vi "Create Plugin Project.vi"(8 "error in":errorcluster, 9 "Custom Device Name":string, 11 "CDEW_MetaDataObj in":refnum<class "NIVS_CDEW_MetaDataObj.lvclass">) -> (0 "error out":errorcluster, 3 "CDEW_MetaDataObj out":refnum<class "NIVS_CDEW_MetaDataObj.lvclass">)   [LabVIEW 2026, in "NIVS_CDEW_MetaDataObj.lvclass"]
uses:
  NIVS_CDEW_MetaDataObj.lvclass
  Types/PluginProjectToolStates.ctl
  NIVS_CDEW_MetaDataObj.lvclass/NIVS_CDEW_MetaDataObj.ctl
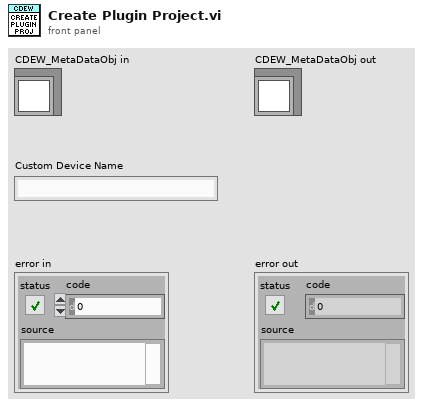
[diagram p1: front panel]
types:
  T1 = typedef "NIVS_CDEW_MetaDataObj.lvclass/PluginProjectToolStates.ctl" = enum16{"CopyAndRenamePluginLVLIB", "CopyAndRenameDeploymentHooksLVLIB", "UpdateProject"}
  T2 = typedef "NIVS_CDEW_MetaDataObj.lvclass/Execution Modes.ctl" = enum16{"Inline HW Interface (Inline-Async API)", "Inline HW Interface", "Inline Timing and Sync"}
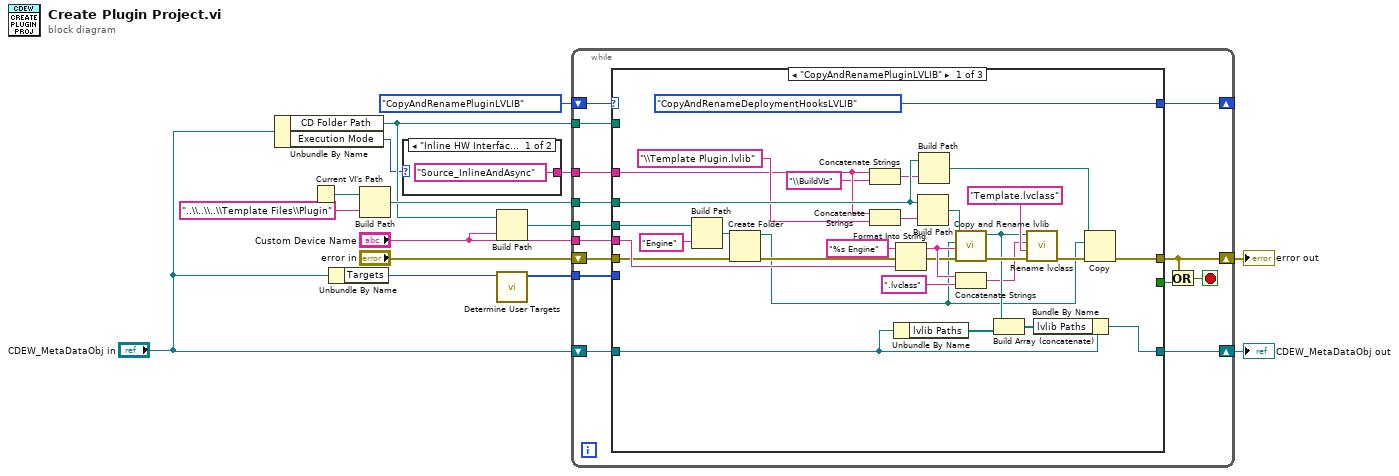
[diagram p0: block diagram]
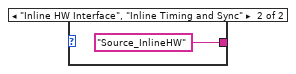
[diagram p2: hidden frame]
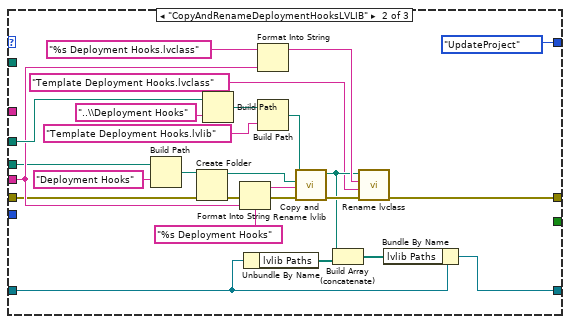
[diagram p3: hidden frame]
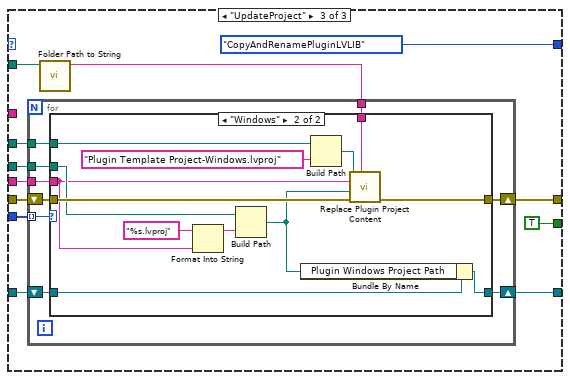
[diagram p4: hidden frame]
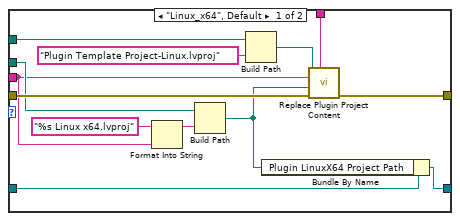
[diagram p5: hidden frame]
diagram:
  n1 = Unbundle By Name("CDEW_MetaDataObj in") -> ("CD Folder Path"=w4:path, "Execution Mode"=w3:T2)
  n2 = Current VI's Path() -> (path=w14:path)
  n3 = Unbundle By Name("CDEW_MetaDataObj in") -> ("Targets"=w5:enum16{"Linux_x64", "Windows", "Both"})
  n4 = Build Path(base path=w14, name or relative path="..\\..\\..\\Template Files\\Plugin") -> (appended path=w12:path)
  n5 = case shown="\"Inline HW Interface (Inline-Async API)\", Default" w3 {
    tunnel: ["Source_InlineAndAsync" ("string") "Source_InlineHW" ("string")] -> w9
    frame "Inline HW Interface (Inline-Async API)", Default {
    }
    frame "Inline HW Interface", "Inline Timing and Sync" {
    }
  }
  n6 = Build Path(base path=w4, name or relative path="Custom Device Name") -> (appended path=w7:path)
  n7 = call "Determine User Targets.vi"("Targets"=w5) -> ("User Configured Targets"=w6:enum16{"Linux_x64", "Windows", "Both"}[])  [unwired: 10 in]
  n8 = while {
    shift-right: [w27] -> _
    shift-left: PluginProjectToolStates."CopyAndRenamePluginLVLIB" ("Enum") -> [w31]
    tunnel: w7 -> [w30]
    tunnel: "Custom Device Name" -> [w29]
    tunnel: w12 -> [w28]
    shift-right: [w25] -> w10
    shift-left: "error in" -> [w26]
    tunnel: w9 -> [w22]
    tunnel: w4 -> [w21]
    tunnel: w6 -> [w20]
    shift-right: [w18] -> w1
    shift-left: "CDEW_MetaDataObj in" -> [w19]
    stop <- w23 stop-if-true
    n9 = case shown="\"CopyAndRenamePluginLVLIB\"" w31 {
      tunnel: w30 -> [w37 w69 w90]
      tunnel: w29 -> [w46 w79 w98]
      tunnel: w28 -> [w57 w87 w96]
      tunnel: [PluginProjectToolStates."CopyAndRenameDeploymentHooksLVLIB" ("Enum") PluginProjectToolStates."UpdateProject" ("Enum") PluginProjectToolStates."CopyAndRenamePluginLVLIB" ("Enum")] -> w27
      tunnel: [_ _ TRUE] -> w24
      tunnel: [w53 w77 w97] -> w25
      tunnel: w26 -> [w34 w71 w94]
      tunnel: w22 -> [w50 _ _]
      tunnel: w21 -> [_ _ w92]
      tunnel: w20 -> [_ _ w91]
      tunnel: w19 -> [w39 w62 w89]
      tunnel: [w40 w63 w88] -> w18
      frame "CopyAndRenamePluginLVLIB" {
        n10 = Build Path(base path=w37, name or relative path="Engine" ("string")) -> (appended path=w33:path)
        n11 = Create Folder(path (use dialog)=w33, error in=w34) -> (created path=w32:path, error out=w35:errorcluster)  [unwired: 1 in, 1 out]
        n12 = Concatenate Strings(w50, "\\BuildVIs" ("format string")) -> (w48:string)
        n13 = Concatenate Strings(w50, "\\Template Plugin.lvlib" ("string")) -> (w51:string)
        n14 = Unbundle By Name(w39) -> ("lvlib Paths"=w42:path[])
        n15 = Format Into String(format string="%s Engine", error in=w35, w46) -> (resulting string=w45:string, error out=w36:errorcluster)  [unwired: 1 in]
        n16 = Build Path(base path=w57, name or relative path=w51) -> (appended path=w59:path)
        n17 = Build Path(base path=w57, name or relative path=w48) -> (appended path=w56:path)
        n18 = call "Copy and Rename lvlib.vi"("error in"=w36, "New lvlib Name"=w45, "Destination Directory Path"=w32, "lvlib Path"=w59) -> ("error out"=w61:errorcluster, "New Library Path"=w54:path)  [unwired: 6 in]
        n19 = Concatenate Strings(w45, ".lvclass" ("format string")) -> (w43:string)
        n20 = Build Array (concatenate)(w54, w42) -> (w41:path[])
        n21 = call "Rename lvclass.vi"("error in"=w61, "Template class name"="Template.lvclass" ("format string"), "New class name"=w43, "lvlib path"=w54) -> ("error out"=w55:errorcluster)  [unwired: 7 in]
        n22 = Bundle By Name(cluster=w39, "lvlib Paths"=w41) -> (w40:refnum<class "NIVS_CDEW_MetaDataObj.lvclass">)
        n23 = Copy(8:w55, 10:w32, 11:w56) -> (0:w53:errorcluster)  [unwired: 2 in, 2 out]
      }
      frame "CopyAndRenameDeploymentHooksLVLIB" {
        n24 = Build Path(base path=w69, name or relative path="Deployment Hooks" ("string")) -> (appended path=w67:path)
        n25 = Create Folder(path (use dialog)=w67, error in=w71) -> (created path=w66:path, error out=w72:errorcluster)  [unwired: 1 in, 1 out]
        n26 = Build Path(base path=w87, name or relative path="..\\Deployment Hooks" ("string")) -> (appended path=w70:path)
        n27 = Format Into String(format string="%s Deployment Hooks", error in=w72, w79) -> (resulting string=w74:string, error out=w73:errorcluster)  [unwired: 1 in]
        n28 = Unbundle By Name(w62) -> ("lvlib Paths"=w65:path[])
        n29 = Format Into String(format string="%s Deployment Hooks.lvclass", w79) -> (resulting string=w84:string)  [unwired: 2 in, 1 out]
        n30 = Build Path(base path=w70, name or relative path="Template Deployment Hooks.lvlib" ("Template class name")) -> (appended path=w81:path)
        n31 = call "Copy and Rename lvlib.vi"("error in"=w73, "New lvlib Name"=w74, "Destination Directory Path"=w66, "lvlib Path"=w81) -> ("error out"=w83:errorcluster, "New Library Path"=w78:path)  [unwired: 6 in]
        n32 = Build Array (concatenate)(w78, w65) -> (w64:path[])
        n33 = call "Rename lvclass.vi"("error in"=w83, "Template class name"="Template Deployment Hooks.lvclass", "New class name"=w84, "lvlib path"=w78) -> ("error out"=w77:errorcluster)  [unwired: 7 in]
        n34 = Bundle By Name(cluster=w62, "lvlib Paths"=w64) -> (w63:refnum<class "NIVS_CDEW_MetaDataObj.lvclass">)
      }
      frame "UpdateProject" {
        n35 = call "Folder Path to String.vi"("CD Folder Path"=w92) -> ("Path as String"=w93:string)  [unwired: 10 in]
        n36 = for {
          tunnel: w98 -> [w103]
          tunnel: w96 -> [w107]
          tunnel: w93 -> [w105]
          shift-right: [w108] -> w97
          shift-left: w94 -> [w106]
          tunnel: w91 -> [w100] mode=indexing
          tunnel: w90 -> [w104]
          shift-right: [w101] -> w88
          shift-left: w89 -> [w102]
          n37 = case shown="\"Windows\"" w100 {
            tunnel: [w121 w134] -> w108
            tunnel: w107 -> [w120 w133]
            tunnel: w106 -> [w117 w130]
            tunnel: w105 -> [w116 w129]
            tunnel: w104 -> [w115 w128]
            tunnel: w103 -> [w112 w125]
            tunnel: w102 -> [w111 w124]
            tunnel: [w110 w123] -> w101
            frame "Linux_x64", Default {
              n38 = Format Into String(format string="%s Linux x64.lvproj", w112) -> (resulting string=w113:string)  [unwired: 2 in, 1 out]
              n39 = Build Path(base path=w115, name or relative path=w113) -> (appended path=w109:path)
              n40 = Build Path(base path=w120, name or relative path="Plugin Template Project-Linux.lvproj" ("Custom Device Name")) -> (appended path=w118:path)
              n41 = Bundle By Name(cluster=w111, "Plugin LinuxX64 Project Path"=w109) -> (w110:refnum<class "NIVS_CDEW_MetaDataObj.lvclass">)
              n42 = call "Replace Plugin Project Content.vi"("CDFolder Path String"=w116, "error in"=w117, "Plugin Project Path"=w109, "Plugin Name"=w112, "Template Project path"=w118) -> ("error out"=w121:errorcluster)  [unwired: 6 in]
            }
            frame "Windows" {
              n43 = Format Into String(format string="%s.lvproj", w125) -> (resulting string=w126:string)  [unwired: 2 in, 1 out]
              n44 = Build Path(base path=w128, name or relative path=w126) -> (appended path=w122:path)
              n45 = Bundle By Name(cluster=w124, "Plugin Windows Project Path"=w122) -> (w123:refnum<class "NIVS_CDEW_MetaDataObj.lvclass">)
              n46 = Build Path(base path=w133, name or relative path="Plugin Template Project-Windows.lvproj" ("Custom Device Name")) -> (appended path=w131:path)
              n47 = call "Replace Plugin Project Content.vi"("CDFolder Path String"=w129, "error in"=w130, "Plugin Project Path"=w122, "Plugin Name"=w125, "Template Project path"=w131) -> ("error out"=w134:errorcluster)  [unwired: 6 in]
            }
          }
        }
      }
    }
    n48 = Or(x=w25, y=w24) -> (x .or. y?=w23:bool)
  }
  "error out" <- w10
  "CDEW_MetaDataObj out" <- w1
